vi "ReachGoal.vi"(8 "error in":errorcluster, 10 "Goal point":T4) -> (0 "error out":errorcluster)   [LabVIEW 2009, in "Main.lvlib"]
doc: "Main subroutine for reach specified point."
uses:
  Main.lvlib
  Drive/Drive_Point.ctl
  MainVariables.lvlib
  NetworkVarTarget.lvlib
  Drive/Drive_Utils.lvlib
  Drive.lvlib
panel:
  out "Objects bottom cords":T1(array[cluster])
  out "Walls":T2(array[cluster])
  out "state out":T3
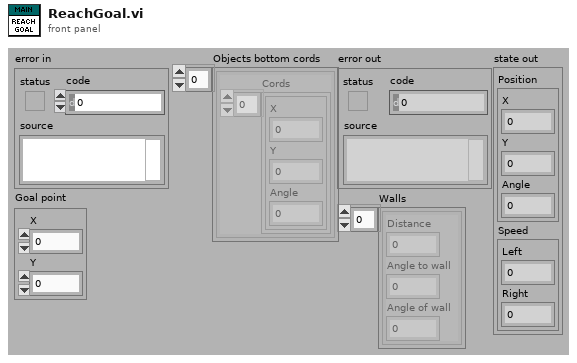
[diagram p1: front panel]
types:
  T1 = cluster{"Cords":cluster{"X":dbl, "Y":dbl, "Angle":dbl}[]}[]
  T2 = cluster{"Distance":dbl, "Angle to wall":dbl, "Angle of wall":dbl}[]
  T3 = cluster{"Position":cluster{"X":dbl, "Y":dbl, "Angle":dbl}, "Speed":cluster{"Left":dbl, "Right":dbl}}
  T4 = typedef "Drive.lvlib/Drive_Point.ctl" = cluster{"X":dbl, "Y":dbl}
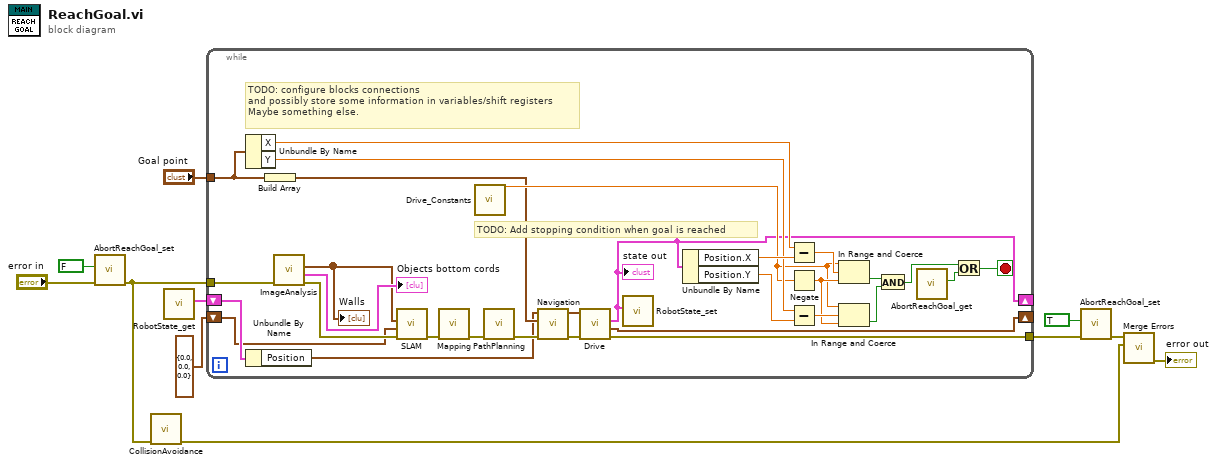
[diagram p0: block diagram]
diagram:
  n1 = call "AbortReachGoal_set.vi"("error in (no error)"="error in", "Abort? (F)"=FALSE) -> ("error out"=w7:errorcluster)  [unwired: 9 in]
  n2 = call "CollisionAvoidance.vi"("error in"=w7) -> ("error out"=w6:errorcluster)  [unwired: 10 in]
  n3 = call "RobotState_get.vi"() -> ("RobotState"=w2:T3)  [unwired: 10 in, 1 out]
  n4 = while {
    tunnel: w7 -> [w41]
    tunnel: [w37] -> w5
    tunnel: "Goal point" -> [w19]
    shift-right: [w17] -> _
    shift-left: w2 -> [w16]
    shift-right: [w13] -> _
    shift-left: cluster{"X":dbl, "Y":dbl, "Angle":dbl} {"X"=0.0, "Y"=0.0, "Angle"=0.0} ("deltaPosition") -> [w12]
    stop <- w32 stop-if-true
    # "TODO: Add stopping condition when goal is reached"
    # "TODO: configure blocks connections\nand possibly store some information in variables/shift registers\nMaybe something else."
    n5 = Unbundle By Name(w19) -> ("X"=w27:dbl, "Y"=w25:dbl)
    n6 = Unbundle By Name(w16) -> ("Position"=w15:cluster{"X":dbl, "Y":dbl, "Angle":dbl})
    n7 = Build Array(w19) -> (w18:T4[])
    n8 = call "ImageAnalysis.vi"("error in"=w41) -> ("error out"=w40:errorcluster, "Objects bottom cords"=→"Objects bottom cords":T1, "Walls"=w14:T2)  [unwired: 8 in]
    "Walls" <- w14
    n9 = call "SLAM.vi"("error in"=w40, "deltaPosition"=w12, "Walls"=w14) -> ("error out"=w39:errorcluster)  [unwired: 7 in, 1 out]
    n10 = call "Mapping.vi"("error in"=w39) -> ("error out"=w35:errorcluster)  [unwired: 10 in]
    n11 = call "Drive_Constants.vi"() -> ("Position accuracy (m)"=w21:dbl)  [unwired: 19 in, 8 out]
    n12 = call "PathPlanning.vi"("error in"=w35) -> ("error out"=w36:errorcluster)  [unwired: 10 in]
    n13 = call "Navigation.vi"("error in"=w36, "Array of path nodes"=w18, "Robot current position"=w15) -> ("error out"=w38:errorcluster, "Movements"=w20:cluster{"Left":dbl, "Right":dbl}[])  [unwired: 7 in]
    n14 = call "Drive.vi"("error in"=w38, "Movements"=w20) -> ("error out"=w37:errorcluster, "deltaPosition"=w13:cluster{"X":dbl, "Y":dbl, "Angle":dbl}, "state out"=w17:T3)  [unwired: 7 in]
    "state out" <- w17
    n15 = call "RobotState_set.vi"("RobotState"=w17) -> ()  [unwired: 10 in, 1 out]
    n16 = Unbundle By Name(w17) -> ("Position.X"=w26:dbl, "Position.Y"=w24:dbl)
    n17 = Subtract(x=w27, y=w26) -> (x-y=w28:dbl)
    n18 = Negate(x=w21) -> (-x=w22:dbl)
    n19 = Subtract(x=w25, y=w24) -> (x-y=w23:dbl)
    n20 = In Range and Coerce(upper limit=w21, x=w28, lower limit=w22) -> (In Range?=w31:bool)  [unwired: 1 out]
    n21 = In Range and Coerce(upper limit=w21, x=w23, lower limit=w22) -> (In Range?=w30:bool)  [unwired: 1 out]
    n22 = And(x=w31, y=w30) -> (x .and. y?=w29:bool)
    n23 = call "AbortReachGoal_get.vi"() -> ("Abort"=w33:bool)  [unwired: 10 in, 1 out]
    n24 = Or(x=w29, y=w33) -> (x .or. y?=w32:bool)
  }
  n25 = call "AbortReachGoal_set.vi"("error in (no error)"=w5, "Abort? (F)"=TRUE) -> ("error out"=w3:errorcluster)  [unwired: 9 in]
  n26 = call <vilib>:"Merge Errors.vi"("error in 2 (no error)"=w6, "error in 1 (no error)"=w3) -> ("error out"=→"error out":errorcluster)  [unwired: 5 in]
